vi "判断节点合法.vi"(11 "节点数组":T1(array[cluster])) -> (3 "合法":bool)   [LabVIEW 2019]
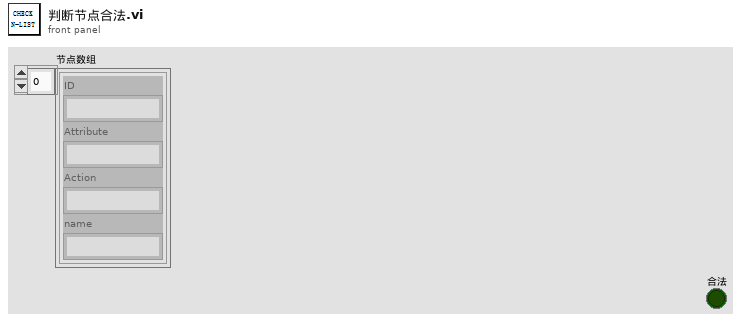
[diagram p1: front panel]
types:
  T1 = cluster{"ID":string, "Attribute":string, "Action":string, "name":string}[]
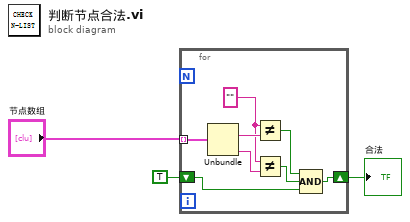
[diagram p0: block diagram]
diagram:
  n1 = for {
    tunnel: "节点数组" -> [w11] mode=indexing
    shift-right: [w5] -> w2
    shift-left: TRUE -> [w4]
    w8 = "" ("x")
    n2 = Unbundle(w11) -> ("Attribute"=w10:string, "name"=w9:string)  [unwired: 2 out]
    n3 = Not Equal?(x=w8, y=w10) -> (x != y?=w7:bool)
    n4 = Not Equal?(x=w8, y=w9) -> (x != y?=w6:bool)
    n5 = Compound Arithmetic op=AND ("复合运算")(w7, w6, w4) -> (w5:bool)
  }
  "合法" <- w2
